vi "Init5Panes.vi"(5 "Horizontal Resizing Pane":u16(ring)=1 items=["left", "middle", "right"], 7 "Vertical Resizing Pane":u16(ring)=1 items=["top", "middle", "bottom"], 8 "error in (no error)":errorcluster, 9 "Pane Sizes Top;Left;Right;Bottom":i32[](array[numeric])=[0, 0, 0, 0], 10 "Path":path) -> (0 "error out":errorcluster, 2 "Panes":T1, 3 "PentaPanesGUI out":refnum<class "PentaPanes.lvclass">)   [LabVIEW 2022 SP3, in "PentaPanesLibrary.lvlib" / "PentaPanes.lvclass"]
doc: "This VI Initializes the PentaPanes object.\n\n\nPath - Path to the VI containing the 5 panes FrontPanel\nPane Sizes - An array of initial sizes of panes\nVertical Resizing Pane - Select the pane to change its height when front panel window height changes\nHorizontal Resizing Pane - Select the pane to change its width when front panel window width changes \nPanes - An output cluster of the panes detected."
uses:
  PentaPanes.lvclass
  PanesCluster.ctl
  PanesOrigin.ctl
  ResizableObject.ctl
  BordersCluster.ctl
  <vilib>/Utility/miscctls.llb/LVBoundsTypeDef.ctl
  PanePosition.ctl
  PentaPanes.lvclass/PentaPanes.ctl
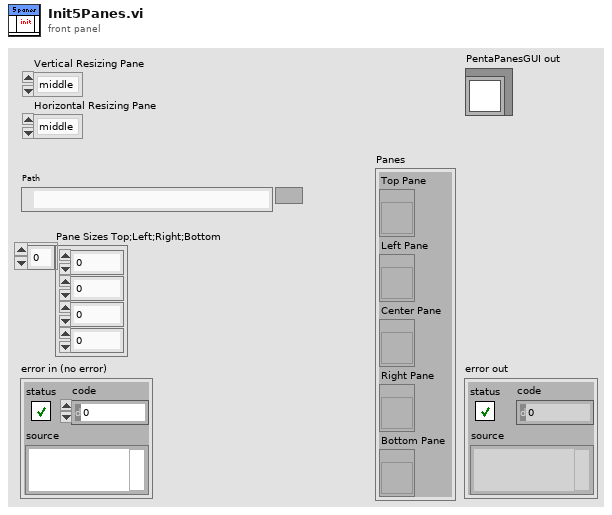
[diagram p1: front panel]
types:
  T1 = typedef "PentaPanesLibrary.lvlib/PentaPanes.lvclass/PanesCluster.ctl" = cluster{"Top Pane":refnum<vi>, "Left Pane":refnum<vi>, "Center Pane":refnum<vi>, "Right Pane":refnum<vi>, "Bottom Pane":refnum<vi>}
  T2 = typedef "PentaPanesLibrary.lvlib/PentaPanes.lvclass/PanesOrigin.ctl" = cluster{"Top Pane Origin":cluster{"X":u32, "Y":u32}, "Left Pane Origin":cluster{"X":u32, "Y":u32}, "Center Pane Origin":cluster{"X":u32, "Y":u32}, "Right Pane Origin":cluster{"X":u32, "Y":u32}, "Bottom Pane Origin":cluster{"X":u32, "Y":u32}}
  T3 = typedef "PentaPanesLibrary.lvlib/PentaPanes.lvclass/ResizableObject.ctl" = cluster{"generic class reference":refnum<vi>, "Label out":string, "Adjust":u16, "Borders":T4, "Minimal":T5, "Class Name out":string, "Class ID out":u32, "Owning Pane out":refnum<vi>, "Borders in Percent(T) or Pixels (F)":bool, "Invisible?":bool, "Force Aspect Ratio?":bool}
  T4 = typedef "PentaPanesLibrary.lvlib/PentaPanes.lvclass/BordersCluster.ctl" = cluster{"Left":i32, "Top":i32, "Right":i32, "Bottom":i32}
  T5 = typedef "LVBoundsTypeDef.ctl" = cluster{"Width":i32, "Height":i32}
  T6 = typedef "PentaPanesLibrary.lvlib/PentaPanes.lvclass/PanePosition.ctl" = u16
  T7 = enum16{"Always On", "Always Off", "Off While Running"}[]
  T8 = typedef "PentaPanesLibrary.lvlib/PentaPanes.lvclass/SplittersCluster.ctl" = cluster{"Top Splitter":refnum<vi>, "Left Splitter":refnum<vi>, "Right Splitter":refnum<vi>, "Bottom Splitter":refnum<vi>}
  T9 = typedef "PentaPanesLibrary.lvlib/PentaPanes.lvclass/SplittersWidthCluster.ctl" = cluster{"Top Splitter":i32, "Left Splitter":i32, "Right Splitter":i32, "Bottom Splitter":i32}
  T10 = typedef "PentaPanesLibrary.lvlib/PentaPanes.lvclass/PanesColors.ctl" = cluster{"Top Color":u32, "Left Color":u32, "Center Color":u32, "Right Color":u32, "Bottom Color":u32}
  T11 = cluster{"Position Integer":T6[], "Position String":string[], "Splitter ref":refnum<vi>[], "Pane ref":refnum<vi>[]}
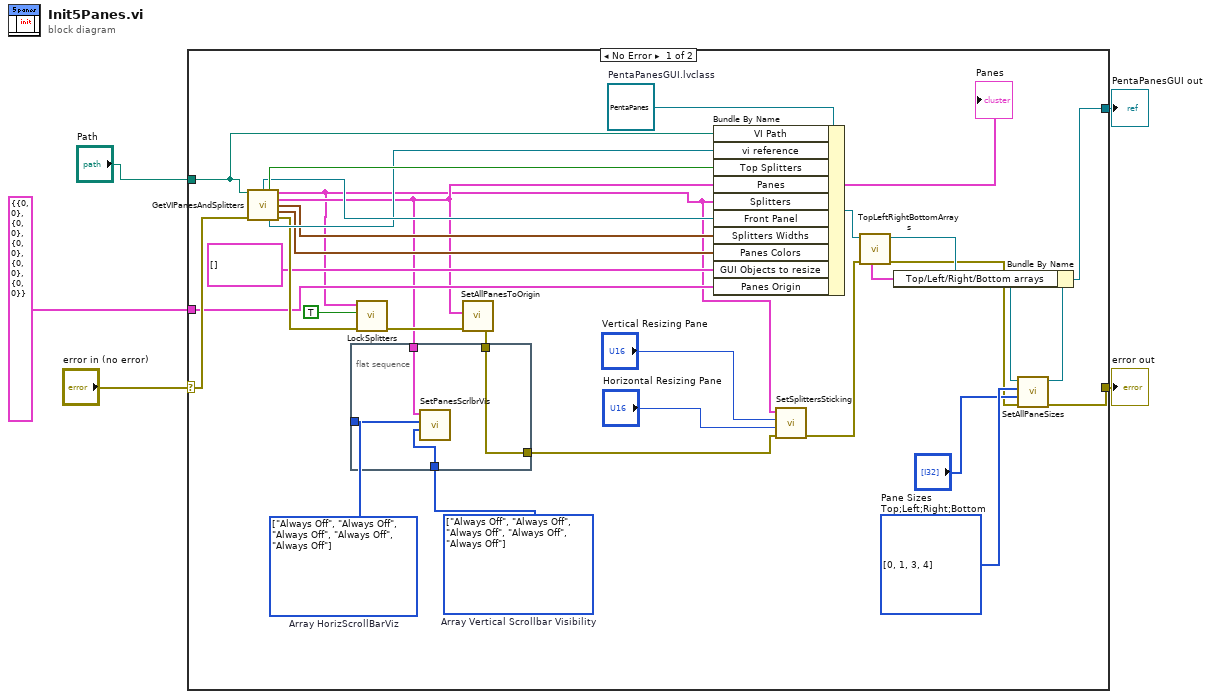
[diagram p0: block diagram]
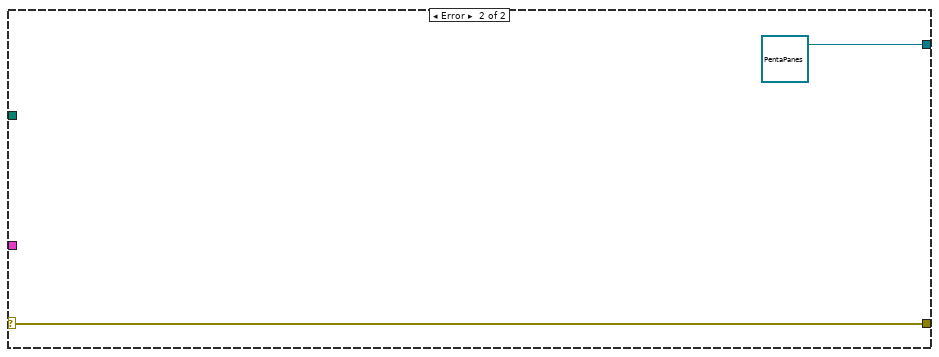
[diagram p2: hidden frame]
diagram:
  n1 = case shown="No Error" "error in (no error)" {
    selector: "error in (no error)" -> [w36 w42]
    tunnel: [w8 w42] -> w4
    tunnel: [w16 refnum<class "PentaPanes.lvclass"> refnum ("PentaPanesGUI.lvclass")] -> w3
    tunnel: "Path" -> [w35 _]
    tunnel: T2 {"Top Pane Origin"={"X"=0, "Y"=0}, "Left Pane Origin"={"X"=0, "Y"=0}, "Center Pane Origin"={"X"=0, "Y"=0}, "Right Pane Origin"={"X"=0, "Y"=0}, "Bottom Pane Origin"={"X"=0, "Y"=0}} ("Panes Origin") -> [w25 _]
    frame No Error {
      w11 = T6[] [0, 1, 3, 4] items=["Top", "Left", "Center", "Right", "Bottom"] ("Pane position array")
      w22 = T7 [enum."Always Off", enum."Always Off", enum."Always Off", enum."Always Off", enum."Always Off"] items=["Always On", "Always Off", "Off While Running"]  # Array Vertical Scrollbar Visibility
      w21 = T7 [enum."Always Off", enum."Always Off", enum."Always Off", enum."Always Off", enum."Always Off"] items=["Always On", "Always Off", "Off While Running"]  # Array HorizScrollBarViz
      w24 = refnum<class "PentaPanes.lvclass"> refnum  # PentaPanesGUI.lvclass
      n2 = call "GetVIPanesAndSplitters.vi"("path"=w35, "error in (no error)"=w36) -> ("Front Panel"=w33:refnum<vi>, "Vertical Splitters On top?"=w34:bool, "Splitters"=w14:T8, "Panes"=w23:T1, "Splitters Widths"=w31:T9, "Colors"=w30:T10, "vi reference"=w32:refnum<vi>, "error out"=w28:errorcluster)  [unwired: 5 in, 1 out]
      "Panes" <- w23
      n3 = flat-sequence {
        tunnel: w23 -> [w40]
        tunnel: w22 -> [w39]
        tunnel: w21 -> [w38]
        tunnel: [w37] -> w6
        tunnel: w7 -> [w37]
        frame #0 {
          n4 = call "SetPanesScrlbrVis.vi"("Array Vertical Scrollbar Visibility"=w39, "Array HorizScrollBarViz"=w38, "Panes"=w40) -> ()  [unwired: 9 in]
        }
      }
      n5 = call "LockSplitters.vi"("error in"=w28, "Splitter Position Locked"=TRUE, "Splitters"=w14) -> ("error out"=w29:errorcluster)  [unwired: 8 in]
      n6 = call "SetAllPanesToOrigin.vi"("error in"=w29, "Panes"=w23) -> ("error out"=w7:errorcluster)  [unwired: 9 in]
      n7 = Bundle By Name(cluster=w24, "VI Path"=w35, "vi reference"=w32, "Top Splitters"=w34, "Panes"=w23, "Splitters"=w14, "Front Panel"=w33, "Splitters Widths"=w31, "Panes Colors"=w30, "GUI Objects to resize"=T3[] [], "Panes Origin"=w25) -> (w18:refnum<class "PentaPanes.lvclass">)
      n8 = call "SetSplittersSticking.vi"("error in (no error)"=w6, "Horizontal Resizing"="Horizontal Resizing Pane", "Vertical Resizing"="Vertical Resizing Pane", "Splitters"=w14) -> ("error out"=w15:errorcluster)  [unwired: 7 in]
      n9 = call "TopLeftRightBottomArrays.vi"("error in (no error)"=w15, "PentaPanesGUI in"=w18) -> ("error out"=w9:errorcluster, "PentaPanesGUI out"=w13:refnum<class "PentaPanes.lvclass">, "Top/Left/Right/Bottom arrays"=w17:T11)  [unwired: 3 in, 4 out]
      n10 = call "SetAllPaneSizes.vi"("error in (no error)"=w9, "Pane Sizes Array"="Pane Sizes Top;Left;Right;Bottom", "Pane position array"=w11, "PentaPanesGUI in"=w13) -> ("error out"=w8:errorcluster, "PentaPanesGUI out"=w12:refnum<class "PentaPanes.lvclass">)  [unwired: 6 in]
      n11 = Bundle By Name(cluster=w12, "Top/Left/Right/Bottom arrays"=w17) -> (w16:refnum<class "PentaPanes.lvclass">)
    }
    frame Error {
    }
  }
  "error out" <- w4
  "PentaPanesGUI out" <- w3
